vi "实验6.vi"() -> ()   [LabVIEW 2017]
panel:
  in  "停止":bool
  out "倒计时":string
  out "指示":bool
  in  "启动":bool
  in  "枚举":enum16{"6秒", "10秒", "20秒"}(ring)
  # "倒计时器"
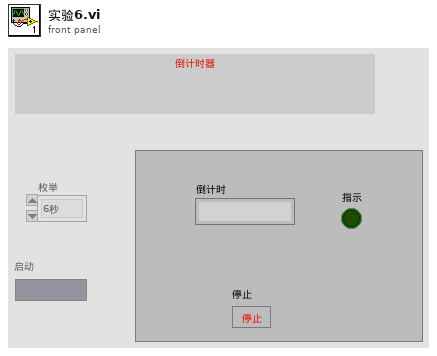
[diagram p1: front panel]
types:
  T1 = enum8{"Enabled", "Disabled", "Disabled and Grayed Out"}
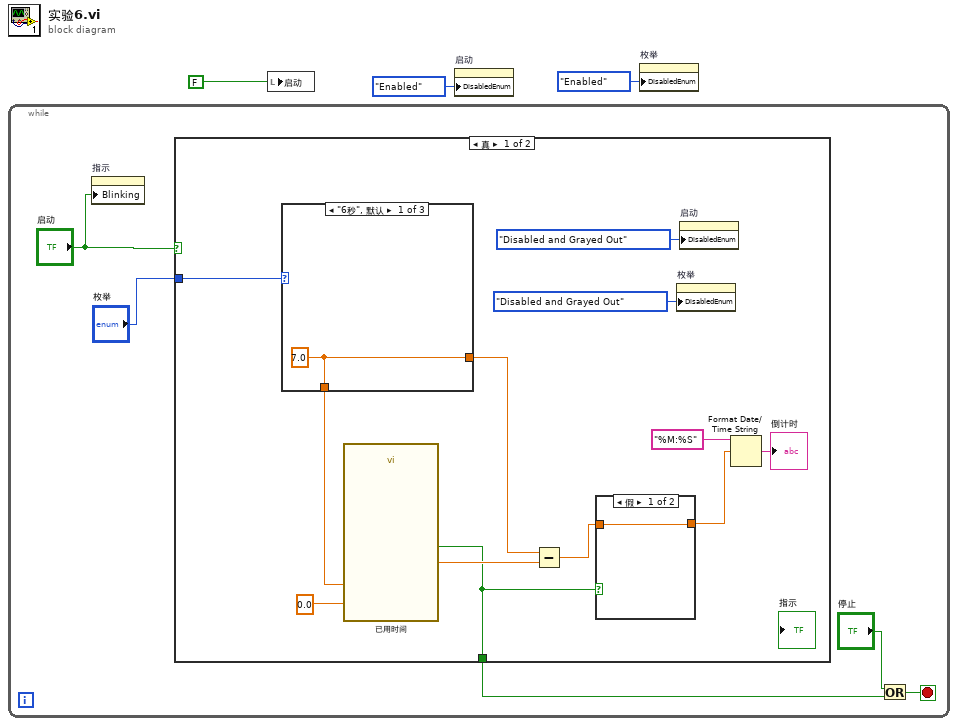
[diagram p0: block diagram]
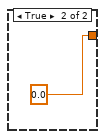
[diagram p2: hidden frame]
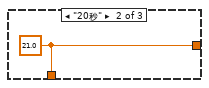
[diagram p3: hidden frame]
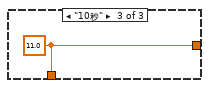
[diagram p4: hidden frame]
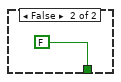
[diagram p5: hidden frame]
diagram:
  n1 = while {
    stop <- w6 stop-if-true
    n2 = property on="指示" class="Bool (严格)"("Blinking"="启动") -> ()  [unwired: 2 in, 2 out]
    n3 = case shown="真" "启动" {
      tunnel: "枚举" -> [w14 _]
      tunnel: [w9 FALSE] -> w5
      frame True {
        n4 = case shown="\"6秒\", 默认" w14 {
          tunnel: [w23 w24 w25] -> w16
          tunnel: [w23 w24 w25] -> w15
          frame "6秒", Default {
            w23 = 7.0 ("y")
          }
          frame "20秒" {
            w24 = 21.0 ("y")
          }
          frame "10秒" {
            w25 = 11.0 ("y")
          }
        }
        n5 = call "已用时间"("Time Target (s)"=w16, "Set Start Time (s)"=0.0) -> ("Elapsed Time (s)"=w18:dbl, "Time has Elapsed"=w9:bool)  [unwired: 10 in, 6 out]
        n6 = Subtract(x=w15, y=w18) -> (x-y=w11:dbl)
        n7 = case shown="假" w9 {
          tunnel: w11 -> [w21 _]
          tunnel: [w21 0.0] -> w10
          frame False {
          }
          frame True {
          }
        }
        n8 = property on="枚举" class="Enum (严格)"("DisabledEnum"=T1."Disabled and Grayed Out" ("禁用")) -> ()  [unwired: 2 in, 2 out]
        n9 = property on="启动" class="Bool (严格)"("DisabledEnum"=T1."Disabled and Grayed Out" ("禁用")) -> ()  [unwired: 2 in, 2 out]
        n10 = Format Date/Time String(time format string (%c)="%M:%S" ("时间格式字符串(%c)"), seconds (now)=w10) -> (date/time string=→"倒计时":string)  [unwired: 1 in]
      }
      frame False {
      }
    }
    n11 = Or(x="停止", y=w5) -> (x .or. y?=w6:bool)
  }
  n12 = local write "启动"(FALSE) -> ()
  n13 = property on="启动" class="Bool (严格)"("DisabledEnum"=T1."Enabled" ("禁用")) -> ()  [unwired: 2 in, 2 out]
  n14 = property on="枚举" class="Enum (严格)"("DisabledEnum"=T1."Enabled" ("禁用")) -> ()  [unwired: 2 in, 2 out]
